vi "Csatornák létrehozása 5.0.vi"(8 "error in":errorcluster, 11 "Analog data in":T3) -> (0 "error out":errorcluster, 3 "Analog data out":T3)   [LabVIEW 2014]
uses:
  Analog data.ctl
  Analog Input Cluster.ctl
  Analog Result Cluster.ctl
panel:
  in  "NI Analog Input":T1 {"Analog Result"."Számolt NTC hõmérséklet" format="%.3g"; "Analog Result"."Semmi 4" format="%.3g"; "Analog Result"."15V" format="%.3g"; "Analog Result"."Semmi 3" format="%.3g"; "Analog Result"."Elvárt NTC ellenállás" format="%.3g"; "Analog Result"."48V" format="%.3g"; "Analog Result"."Hõmérséklet" format="%.3g"; "Analog Result"."Szigetelési ellenállás" format="%.3g"; "Analog Result"."NTC ellenállás" format="%.3g"; "Analog Result"."Szenzor ellenállás" format="%.3g"}
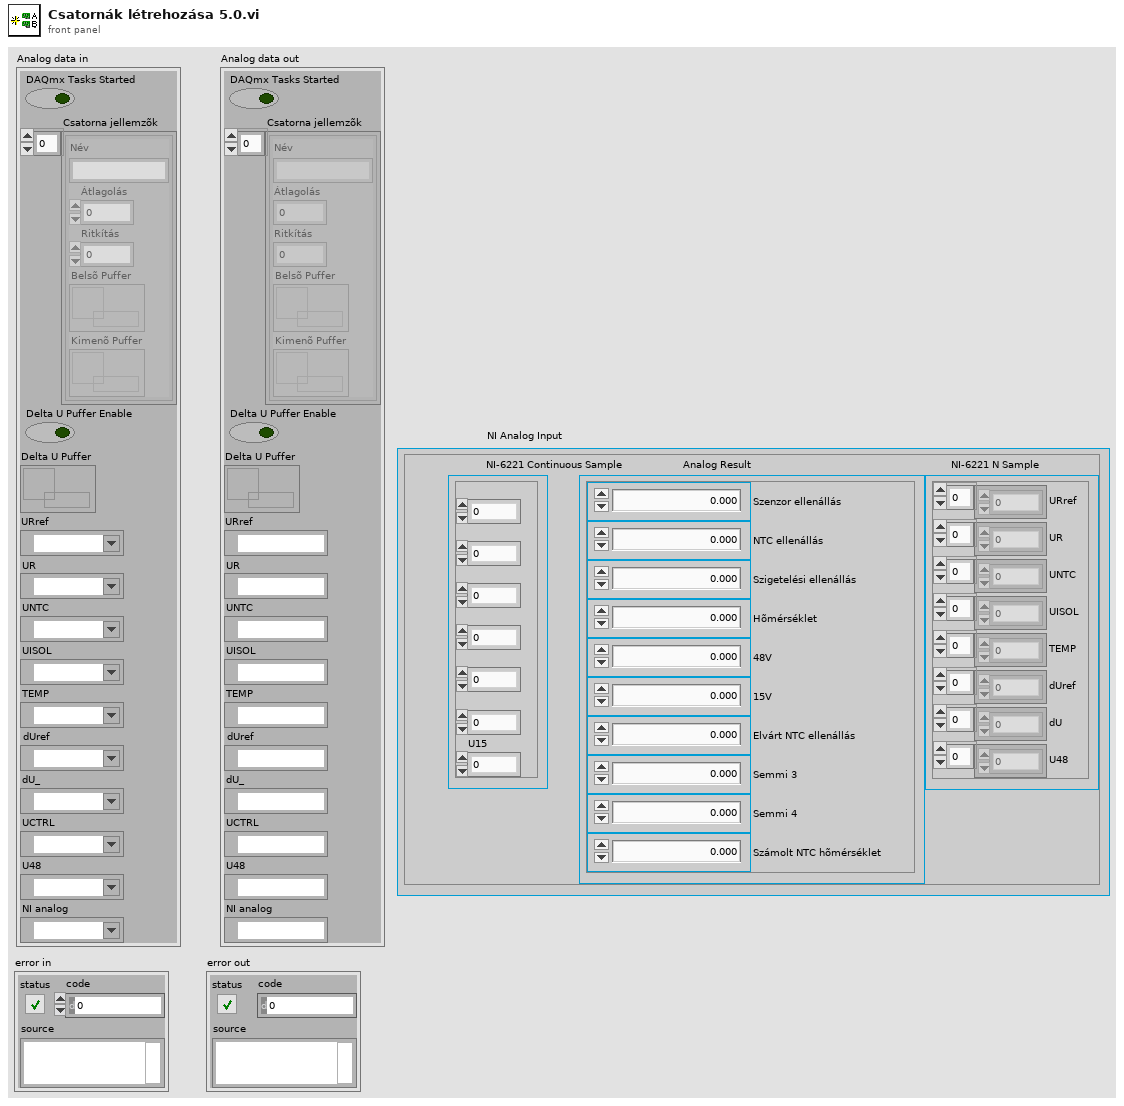
[diagram p1: front panel]
types:
  T1 = typedef "Analog Input Cluster.ctl" = cluster{"NI-6221 Continuous Sample":cluster{"Sensor":dbl, "Uref":dbl, "Temperature":dbl, "Uisol":dbl, "NTC":dbl, "U48":dbl, "U15":dbl}, "Analog Result":T2, "NI-6221 N Sample":cluster{"URref":dbl[], "UR":dbl[], "UNTC":dbl[], "UISOL":dbl[], "TEMP":dbl[], "dUref":dbl[], "dU":dbl[], "U48":dbl[]}}
  T2 = typedef "Analog Result Cluster.ctl" = cluster{"Szenzor ellenállás":dbl, "NTC ellenállás":dbl, "Szigetelési ellenállás":dbl, "Hõmérséklet":dbl, "48V":dbl, "15V":dbl, "Elvárt NTC ellenállás":dbl, "Semmi 3":dbl, "Semmi 4":dbl, "Számolt NTC hõmérséklet":dbl}
  T3 = typedef "Analog data.ctl" = cluster{"DAQmx Tasks Started":bool, "Csatorna jellemzõk":T4[], "Delta U Puffer Enable":bool, "Delta U Puffer":refnum<queue>, "URref":refnum<k21>, "UR":refnum<k21>, "UNTC":refnum<k21>, "UISOL":refnum<k21>, "TEMP":refnum<k21>, "dUref":refnum<k21>, "dU_":refnum<k21>, "UCTRL":refnum<k21>, "U48":refnum<k21>, "NI analog":refnum<k21>}
  T4 = typedef "Csatorna jellemzõk.ctl" = cluster{"Név":string, "Átlagolás":i32, "Ritkítás":i32, "Belsõ Puffer":refnum<queue>, "Kimenõ Puffer":refnum<queue>}
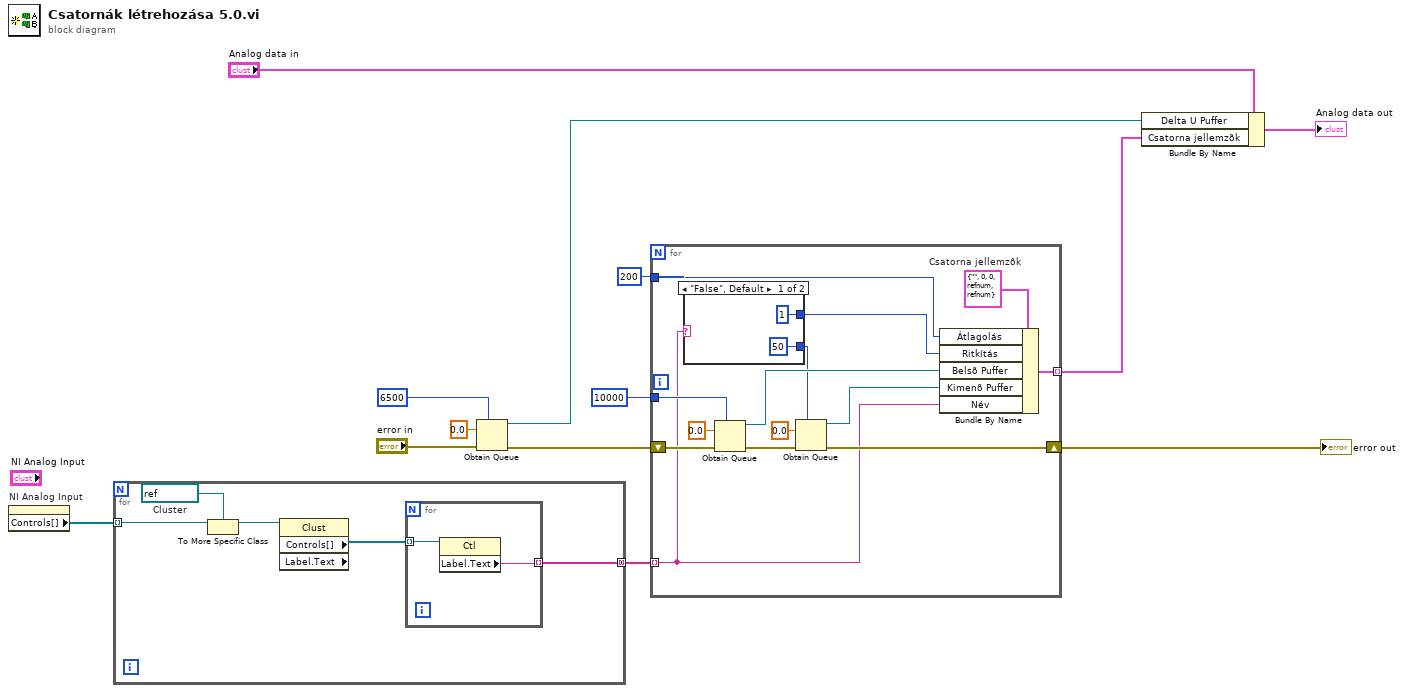
[diagram p0: block diagram]
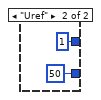
[diagram p2: hidden frame]
diagram:
  n1 = property on="NI Analog Input" class="Clust (strict)"() -> ("Controls[]"=w3:refnum<vi>[])  [unwired: 2 in, 2 out]
  n2 = for {
    tunnel: w3 -> [w15] mode=indexing
    tunnel: [w14] -> w2 mode=concatenating
    w18 = refnum<vi> refnum  # Cluster
    n3 = To More Specific Class(target class=w18, reference=w15) -> (specific class reference=w17:refnum<vi>)  [unwired: 1 in, 1 out]
    n4 = property class="Clust" props=["Controls[]", "Label", "Text"](reference=w17) -> ("Controls[]"=w16:refnum<vi>[])  [unwired: 1 in, 3 out]
    n5 = for {
      tunnel: w16 -> [w20] mode=indexing
      tunnel: [w19] -> w14 mode=indexing
      n6 = property class="Ctl"(reference=w20) -> ("Label.Text"=w19:string)  [unwired: 1 in, 2 out]
    }
  }
  n7 = Obtain Queue(max queue size (-1, unlimited)=6500, element data type=0.0, error in (no error)="error in") -> (queue out=w4:refnum<queue>, error out=w1:errorcluster)  [unwired: 2 in, 1 out]
  n8 = for {
    tunnel: 200 -> [w29]
    tunnel: 10000 -> [w33]
    tunnel: [w31] -> w6 mode=indexing
    shift-right: [w30] -> w11
    shift-left: w1 -> [w24]
    tunnel: w2 -> [w23] mode=indexing
    w34 = T4 {"Név"="", "Átlagolás"=0, "Ritkítás"=0, "Belsõ Puffer"=refnum, "Kimenõ Puffer"=refnum}  # Csatorna jellemzõk
    n9 = case shown="\"False\", Default" w23 {
      tunnel: [50 ("Méret") 50 ("Méret dU")] -> w22
      tunnel: [1 ("Ritkítás") 1 ("Ritkítás dU")] -> w21
      frame "False", Default {
      }
      frame "Uref" {
      }
    }
    n10 = Obtain Queue(max queue size (-1, unlimited)=w33, element data type=0.0, error in (no error)=w24) -> (queue out=w26:refnum<queue>, error out=w27:errorcluster)  [unwired: 2 in, 1 out]
    n11 = Obtain Queue(max queue size (-1, unlimited)=w22, element data type=0.0, error in (no error)=w27) -> (queue out=w25:refnum<queue>, error out=w30:errorcluster)  [unwired: 2 in, 1 out]
    n12 = Bundle By Name(cluster=w34, "Átlagolás"=w29, "Ritkítás"=w21, "Belsõ Puffer"=w26, "Kimenõ Puffer"=w25, "Név"=w23) -> (w31:T4)
  }
  "error out" <- w11
  n13 = Bundle By Name(cluster="Analog data in", "Delta U Puffer"=w4, "Csatorna jellemzõk"=w6) -> (→"Analog data out":T3)
